vi "Refnum Set.vi"(8 "error in (no error)":errorcluster, 10 "refnum name":string, 11 "Nav6DevRef":T1) -> (0 "error out":errorcluster)   [LabVIEW 2013, in "Nav6.lvlib"]
uses:
  Nav6.lvlib
  Nav6DevRef.ctl
  <vilib>/Rock Robotics/WPI/SerialPort/WPI_SerialPortRef.ctl
  Nav6Mode.ctl
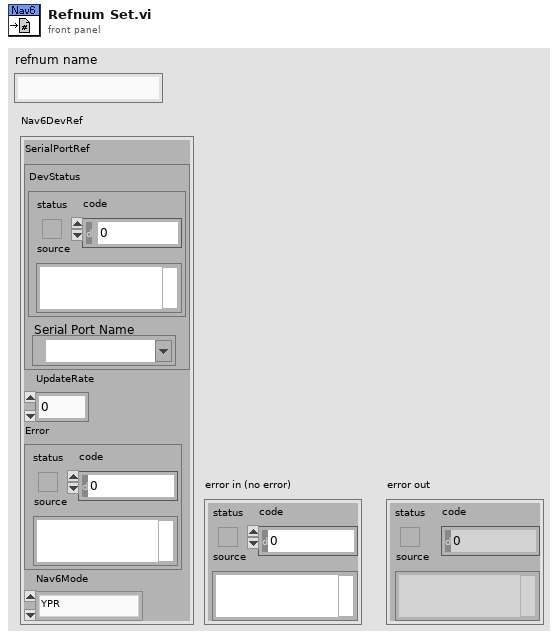
[diagram p1: front panel]
types:
  T1 = typedef "Nav6.lvlib/Nav6DevRef.ctl" = cluster{"SerialPortRef":T2, "UpdateRate":u8, "Error":errorcluster, "Nav6Mode":T3}
  T2 = typedef "WPI_SerialPortRef.ctl" = cluster{"DevStatus":errorcluster, "Serial Port Name":refnum<visa-resource-name>}
  T3 = typedef "Nav6.lvlib/Nav6Mode.ctl" = enum16{"YPR", "Gyro", "Quaternion"}
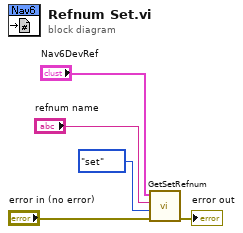
[diagram p0: block diagram]
diagram:
  n1 = call "GetSetRefnum.vi"("error in (no error)"="error in (no error)", "menu"=enum16{"set", "get", "delete"}."set", "refnum name"="refnum name", "Nav6DevRef"="Nav6DevRef") -> ("error out"=→"error out":errorcluster)  [unwired: 6 in, 1 out]
